vi "GUI_HPD_TelescopeStage.vi"() -> ()   [LabVIEW 2013]
uses:
  shared programs/GUI_Template/GUI_master/tcp_new_data_event.ctl
  shared programs/GUI_Template/GUI_master/tcp new data cluster.ctl
panel:
  in  "highspeed::1":dbl=0.001 caption="Speed" min=1000.0 max=6000000.0 format="%_4p"
  in  "stop":bool
  in  "position::1":dbl=0.001 caption="Position" min=0.0 max=550.0 step=1.0 format="%_4p"
  in  "GUIdevice 1":string="HPDTelescopeStage"
  out "tcp data event":T1
  out "error IO 2":errorcluster
  # "HPD Telescope Stage"
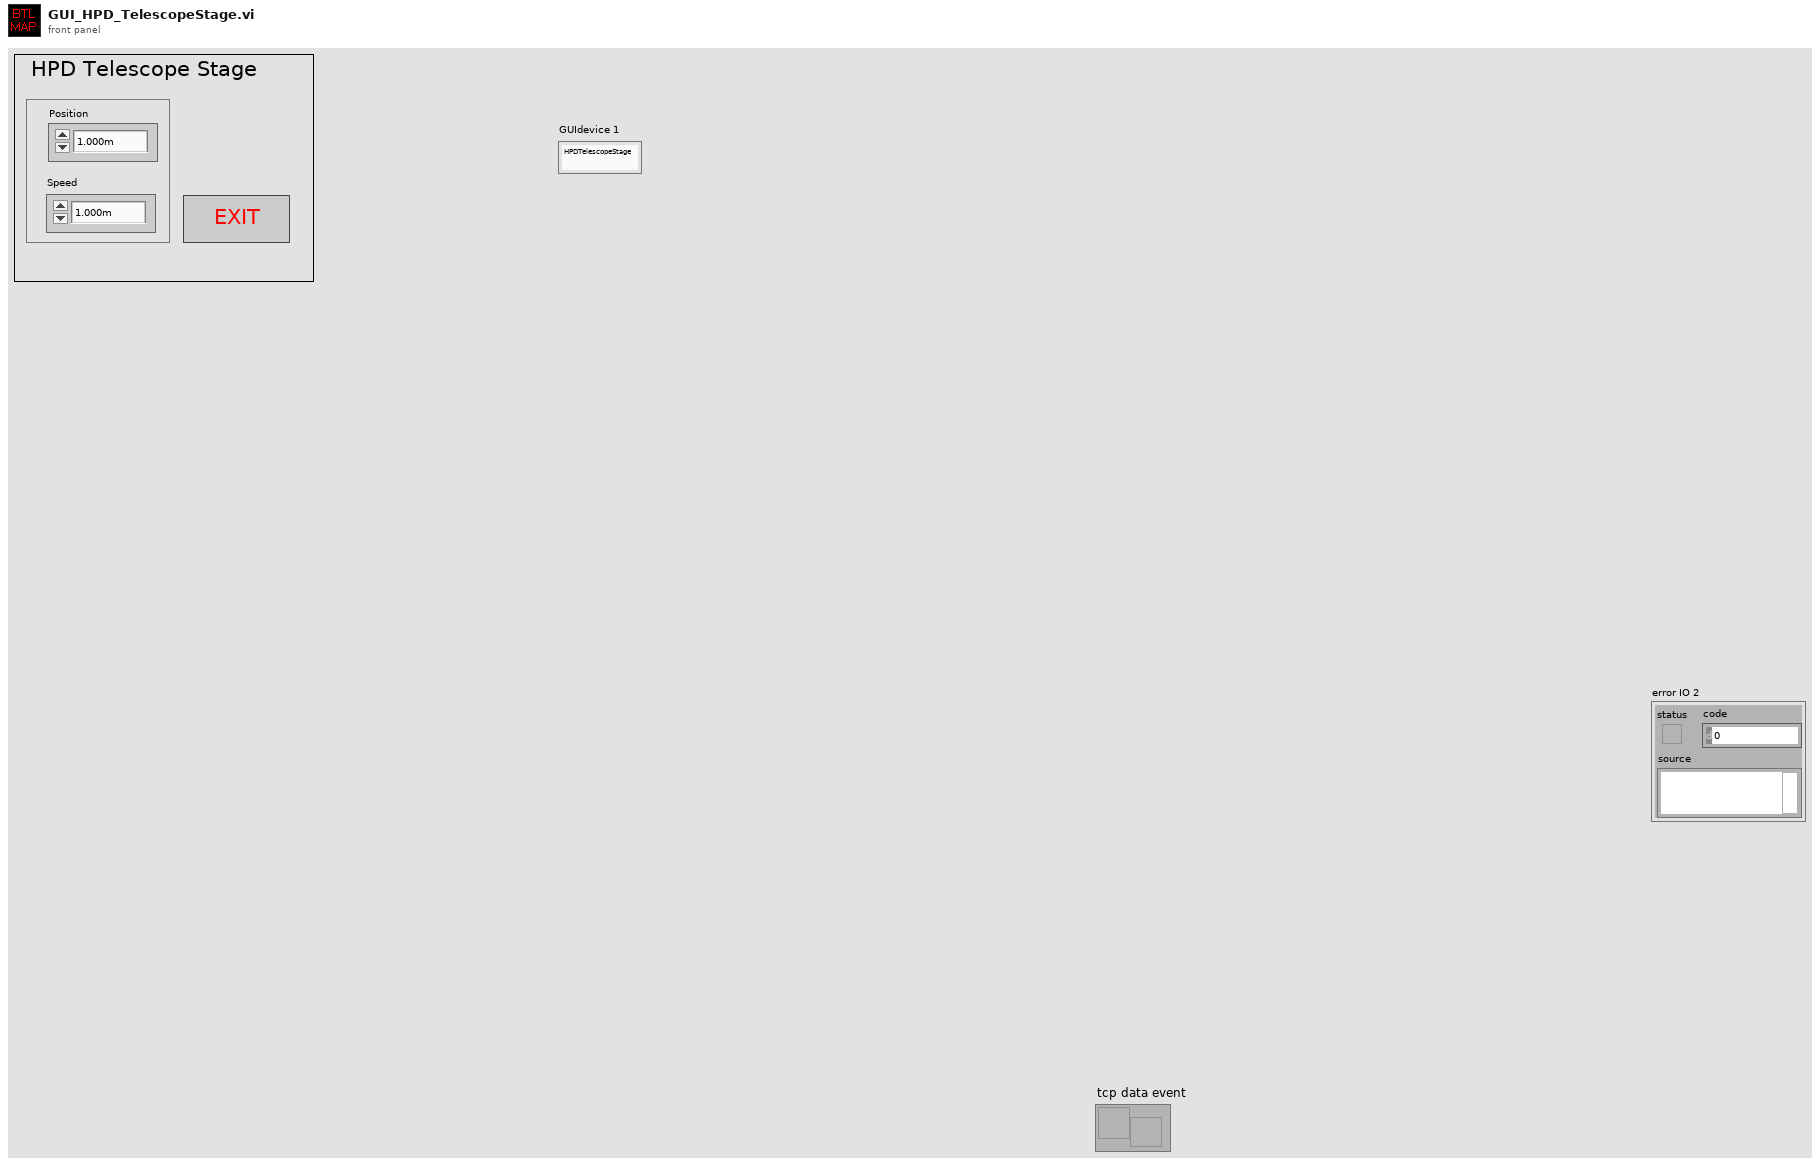
[diagram p1: front panel]
types:
  T1 = typedef "tcp_new_data_event.ctl" = refnum<user-event>
  T2 = typedef "tcp new data cluster.ctl" = cluster{"EventEnum":enum16{"new data", "connection status update"}, "Device name":string}
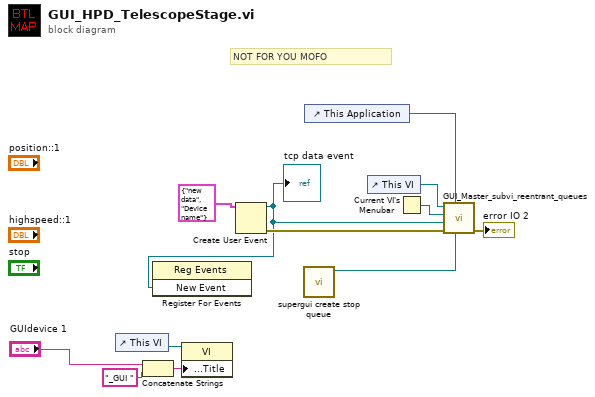
[diagram p0: block diagram]
diagram:
  # "NOT FOR YOU MOFO"
  n1 = control-ref of="This VI"() -> (w4:refnum<vi>)
  n2 = Concatenate Strings("GUIdevice 1", "_GUI ") -> (w3:string)
  n3 = property class="VI"(reference=w4, "Front Panel.Title"=w3) -> ()  [unwired: 1 in, 2 out]
  n4 = Create User Event(user event datatype=T2 {"EventEnum"=enum."new data", "Device name"="Device name"} ("New Event")) -> (user event=w8:refnum<user-event>, error out=w9:errorcluster)  [unwired: 1 in]
  "tcp data event" <- w8
  n5 = register-events(w8) -> ()  [unwired: 2 in, 2 out]
  n6 = call "supergui create stop queue.vi"() -> ("STOP Queue out"=w5:refnum<queue>)  [unwired: 11 in]
  n7 = control-ref of="This Application"() -> (w6:refnum<vi>)
  n8 = control-ref of="This VI"() -> (w7:refnum<vi>)
  n9 = Current VI's Menubar() -> (w11:refnum<k9>)
  n10 = call "GUI_Master_subvi_reentrant_queues.vi"("STOP Queue in"=w5, "This Application"=w6, "error in (no error)"=w9, "tcp data event"=w8, "Caller menu reference"=w11, "Caller VI ref"=w7) -> ("error out"=→"error IO 2":errorcluster)  [unwired: 5 in]
